vi "Publish.vi"(8 "error in (no error)":errorcluster, 9 "Message Priority (Normal)":T1=enum."Normal", 10 "Message":refnum<class "Message.lvclass">, 11 "Publisher in":refnum<class "Publisher.lvclass">) -> (0 "error out":errorcluster, 1 "Callers found?":bool, 3 "Publisher out":refnum<class "Publisher.lvclass">)   [LabVIEW 2020, in "Publisher.lvlib" / "Publisher.lvclass"]
doc: "Publish to subscribers."
uses:
  Publisher.lvclass
  PPL/HDH.Actor Framework.Core.Actor.lvlibp/1abvi3w/vi.lib/ActorFramework/Message/Message.lvclass
  PPL/HDH.Actor Framework.Core.Actor.lvlibp/1abvi3w/vi.lib/ActorFramework/Message Enqueuer/Message Priority.ctl
  Messages/Data Msg/Data Msg.lvclass
  Publisher.lvclass/Publisher.ctl
  PPL/HDH.Actor Framework.Core.Actor.lvlibp/1abvi3w/vi.lib/ActorFramework/Message Enqueuer/Message Enqueuer.lvclass
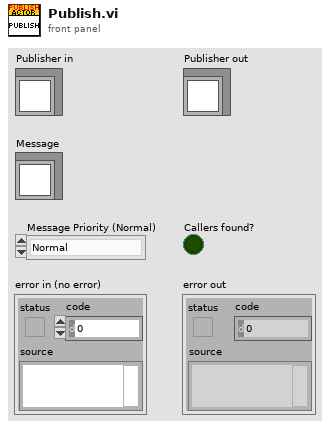
[diagram p1: front panel]
types:
  T1 = typedef "HDH.Actor Framework.Core.Actor.lvlibp/Message Enqueuer.lvclass/Message Priority.ctl" = enum16{"Low", "Normal", "High"}
  T2 = typedef "Publisher.lvlib/Publisher.lvclass/Ctl_Subscription Element.ctl" = cluster{"Object":refnum<class>, "Enqueuers":refnum<class "Message Enqueuer.lvclass">[]}
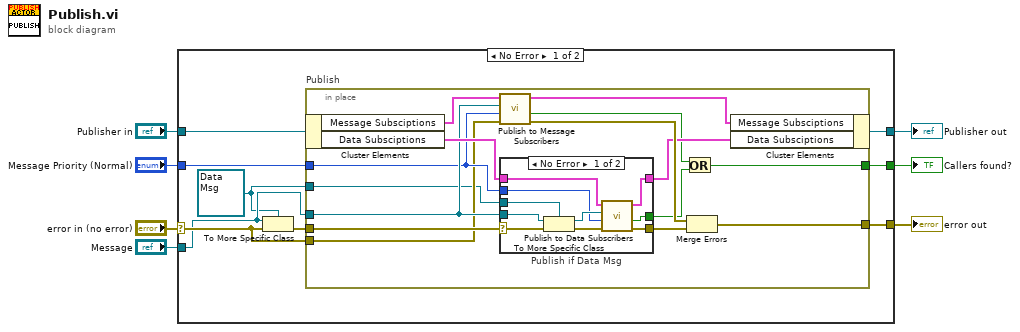
[diagram p0: block diagram]
diagram:
  n1 = case shown="No Error" "error in (no error)" {
    selector: "error in (no error)" -> [w15 w44]
    tunnel: [w12 w44] -> w6
    tunnel: [w13 w43] -> w4
    tunnel: "Publisher in" -> [w16 w43]
    tunnel: "Message" -> [w14 _]
    tunnel: "Message Priority (Normal)" -> [w11 _]
    tunnel: [w8 _] -> w1
    frame No Error {
      w9 = refnum<class "Data Msg.lvclass"> refnum ("Publisher.lvlib:Data Msg.lvclass")
      n2 = To More Specific Class(target class=w9, reference=w14, error in=w15) -> (error out=w10:errorcluster)  [unwired: 1 out]
      n3 = in-place "Publish" {
        in-place-border: [w23] -> w12
        in-place-border: w11 -> [w24]
        in-place-border: w14 -> [w25]
        in-place-border: w15 -> [w21]
        in-place-border: w10 -> [w28]
        in-place-border: w9 -> [w20]
        in-place-border: [w17] -> w8
        n4 = in-place-cluster #1(w16) -> ("Message Subsciptions"=w29:T2[], "Data Subsciptions"=w26:T2[])
        n5 = call "Publish to Message Subscribers.vi"("error in (no error)"=w21, "Message Priority (Normal)"=w24, "Message in"=w25, "Message Subsciptions in"=w29) -> ("error out"=w30:errorcluster, "Callers found?"=w19:bool, "Subsciptions out"=w31:T2[])  [unwired: 5 in]
        n6 = case "Publish if Data Msg" shown="No Error" w28 {
          selector: w28 -> [w40 _]
          tunnel: [w34 w42] -> w27
          tunnel: w26 -> [w38 w42]
          tunnel: w25 -> [w41 _]
          tunnel: w24 -> [w35 _]
          tunnel: [w33 _] -> w22
          tunnel: w20 -> [w39 _]
          tunnel: [w32 _] -> w18
          frame No Error {
            n7 = To More Specific Class(target class=w39, reference=w41, error in=w40) -> (specific class reference=w37:refnum<class "Data Msg.lvclass">, error out=w36:errorcluster)
            n8 = call "Publish to Data Subscribers.vi"("error in (no error)"=w36, "Message Priority (Normal)"=w35, "Data Msg in"=w37, "Data Subsciptions in"=w38) -> ("error out"=w33:errorcluster, "Callers found?"=w32:bool, "Subsciptions out"=w34:T2[])  [unwired: 5 in]
          }
          frame Error {
          }
        }
        n9 = Or(x=w19, y=w18) -> (x .or. y?=w17:bool)
        n10 = Merge Errors(w30, w22) -> (w23:errorcluster)
        n11 = in-place-cluster #1("Message Subsciptions"=w31, "Data Subsciptions"=w27) -> (w13:refnum<class "Publisher.lvclass">)
      }
    }
    frame Error {
    }
  }
  "error out" <- w6
  "Publisher out" <- w4
  "Callers found?" <- w1
